vi "ErrorViewer.Init.vi"(6 "JQMHStartup in":refnum<class "ModuleStartup.lvclass">, 8 "error in (no error)":errorcluster, 11 "ErrorViewer in":refnum<class "ErrorViewer.lvclass">) -> (0 "error out":errorcluster, 1 "StartupParams":variant, 2 "Requests":T1, 3 "Module":refnum<class "ErrorViewer.lvclass">, 4 "JQMHStartup out":refnum<class "ModuleStartup.lvclass">, 5 "StandardRequests":refnum<event-registration>, 7 "External Start?":bool)   [LabVIEW 2024, in "ErrorViewer.lvclass"]
uses:
  ErrorViewer.lvclass
  C:/Git/JA/JQMH/RQMHCore/ModuleCore/Module.lvclass
  RQMHCore/Startup/ModuleStartup.lvclass
  RQMHCore/ErrorReporting/Record/LogRecord.lvclass
  ErrorViewer.lvclass/ErrorViewer.ctl
  RQMHCore/Shared/ModuleShared.lvlib
  RQMHCore/ModuleCore/StopEventArgs.ctl
  RQMHCore/ModuleCore/Module.lvclass
  RQMHCore/ModuleCore/StandardRequests.ctl
  RQMHCore/ModuleCore/Show Front Panel--Args.ctl
  RQMHCore/ModuleCore/Hide Front Panel.ctl
  RQMHCore/ModuleCore/Show Block Diagram.ctl
  RQMHCore/ModuleCore/Hide Block Diagram--Args.ctl
  RQMHCore/ModuleCore/Reply.ctl
  RQMHCore/ModuleCore/InitialiseArgs.ctl
  Do Something Args.ctl
  Request Events--cluster.ctl
  InjectLogEvent.ctl
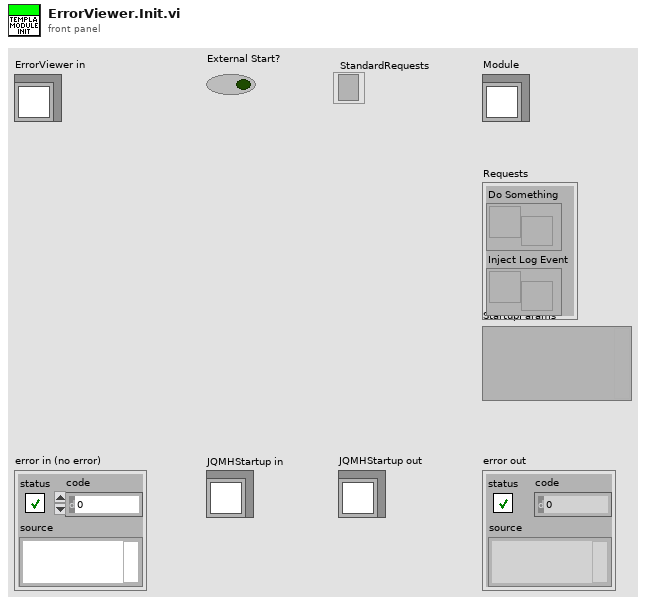
[diagram p1: front panel]
types:
  T1 = typedef "ErrorViewer.lvclass/Request Events--cluster.ctl" = cluster{"Do Something":refnum<user-event>, "Inject Log Event":refnum<user-event>}
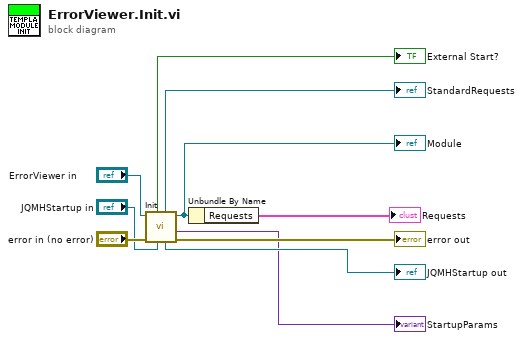
[diagram p0: block diagram]
diagram:
  n1 = call "Init.vi"("JQMHStartup.lvclass"="JQMHStartup in", "error in (no error)"="error in (no error)", "JQMHCore.lvclass"="ErrorViewer in") -> ("error out"=→"error out":errorcluster, "StartupParams"=→"StartupParams":variant, "JQMHCore out"=w10:refnum<class "ErrorViewer.lvclass">, "JQMHStartup out"=→"JQMHStartup out":refnum<class "ModuleStartup.lvclass">, "Event Registration Refnum"=→"StandardRequests":refnum<event-registration>, "External Start?"=→"External Start?":bool)  [unwired: 3 in]
  "Module" <- w10
  n2 = Unbundle By Name(w10) -> ("Requests"=→"Requests":T1)
